vi "test Duplicate.vi"(8 "error in (no error)":errorcluster, 11 "TestCase In":refnum<class "Data Manipulation Tests.lvclass">) -> (0 "error out":errorcluster, 3 "TestCase Out":refnum<class "Data Manipulation Tests.lvclass">)   [LabVIEW 2017, in "Pointer Tests.lvlib" / "Data Manipulation Tests.lvclass"]
uses:
  Data Manipulation Tests.lvclass
  Source/Classes/Pointer/Pointer.lvclass/Pointer.ctl
  Source/Classes/Pointer/Public/New/New (4B).vi
  Source/Classes/Pointer/Public/Write/Write (1D I32).vi
  Source/Classes/Pointer/Private/Allocate.vi
  Source/Classes/Pointer/Public/Write (No Check)/Write (No Check 1D I32).vi
  Source/Classes/Pointer/Protected/Parameter Checking/Check Null Pointer.vi
  Source/Classes/Pointer/Protected/Parameter Checking/Check Subset (Power of 2).vi
  Source/Classes/Pointer/API/Accessors/Get Size.vi
  Source/Classes/Pointer/API/Copy All Pointer Data.vi
  Source/Classes/Pointer/Public/New/New (1B).vi
  Source/Classes/Pointer/Protected/Errors.vi
  Source/Classes/Pointer/Protected/Error VIs/Size Mismatch.vi
  Source/Classes/Pointer/API/Read Pointer Data.vi
  Source/Classes/Pointer/Public/Read/Read (1D U8).vi
  Source/Classes/Pointer/Private/Deallocate.vi
  Source/Classes/Pointer/API/Accessors/Set Address.vi
  Source/Classes/Pointer/API/Accessors/Set Size.vi
  Source/Classes/Pointer/Private/Set Internal.vi
  Source/Classes/Pointer/API/Accessors/Get Address.vi
  Source/Classes/Pointer/Protected/Error VIs/Null Pointer.vi
  Source/Classes/Pointer/Protected/Error VIs/Out of Bounds.vi
  Source/Classes/Pointer/Private/Count to Size.vi
  Source/Classes/Pointer/API/Copy Pointer Data.vi
  Source/Classes/Pointer/Protected/Error Building/Create Error.vi
  Source/VIs/Write String into Source.vi
  Source/VIs/Write Number into Source.vi
  Source/VIs/VIs for Poly/Write U64 into Source.vi
  Source/Classes/Pointer/Public/Read (No Check)/Read (No Check 1D U8).vi
  Source/Classes/Pointer/Protected/Get Internal.vi
  Source/Classes/Pointer/Protected/Error VIs/Zone.vi
  Source/Classes/Pointer/Protected/Error Building/Write Pointer Size.vi
  Source/Classes/Pointer/Public/Copy (No Check).vi
  Source/Classes/Pointer/Protected/Parameter Checking/Check Subset.vi
  Source/Constants/Constants.vi
  Source/Constants/Library Name.vi
  Source/Classes/Pointer/Protected/Error Building/Get Error Info.vi
  Source/VIs/Create Error Cluster.vi
  Source/VIs/VIs for Poly/Create Error Cluster (256B).vi
  Source/VIs/Set Error Status.vi
  Source/VIs/Set Error Code.vi
  Source/VIs/Set Error Source.vi
  Source/Classes/Pointer/Pointer.lvclass
  <vilib>/addons/_JKI Toolkits/VI Tester/TestCase.llb/TestCase.lvclass
  C:/Program Files (x86)/National Instruments/LabVIEW 2017/vi.lib/addons/_JKI Toolkits/VI Tester/TestCase.llb/TestCase.lvclass
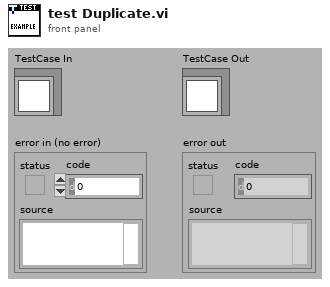
[diagram p1: front panel]
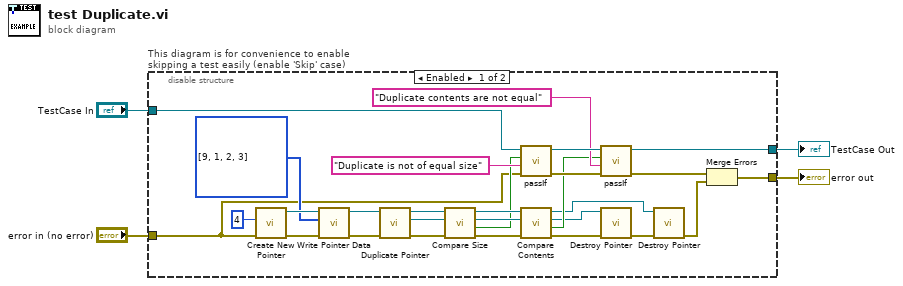
[diagram p0: block diagram]
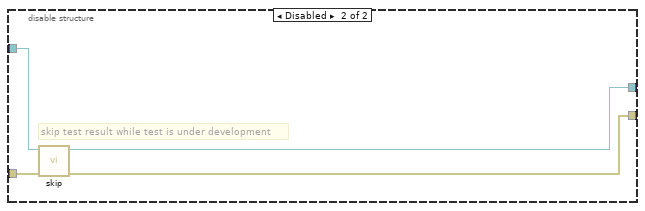
[diagram p2: hidden frame]
diagram:
  n1 = disable-structure "This diagram is for convenience to enable skipping a test easily (enable 'Skip' case)" shown="Enabled" {
    disable-tunnel: "TestCase In" -> [w30 w36]
    disable-tunnel: [w27 w34] -> w1
    disable-tunnel: [w11 w35] -> w3
    disable-tunnel: "error in (no error)" -> [w9 w33]
    frame Enabled {
      n2 = call-poly "Create New Pointer.vi"("error in (no error)"=w9, "count (1)"=u64 4) -> ("error out"=w15:errorcluster, "Pointer"=w32:refnum<class "Pointer.lvclass">)  [unwired: 8 in]
      n3 = call-poly "Write Pointer Data.vi"("error in (no error)"=w15, "buffer in"=i32[] [9, 1, 2, 3] ("count (1)"), "Pointer in"=w32) -> ("error out"=w14:errorcluster, "Pointer out"=w16:refnum<class "Pointer.lvclass">)  [unwired: 5 in, 2 out]
      n4 = call "Duplicate Pointer.vi"("error in (no error)"=w14, "Pointer in"=w16) -> ("error out"=w23:errorcluster, "new duplicate Pointer"=w20:refnum<class "Pointer.lvclass">, "Pointer out"=w24:refnum<class "Pointer.lvclass">)  [unwired: 7 in]
      n5 = call "Compare Size.vi"("error in (no error)"=w23, "Pointer b in"=w20, "Pointer a in"=w24) -> ("error out"=w21:errorcluster, "equal size?"=w18:bool, "Pointer b out"=w19:refnum<class "Pointer.lvclass">, "Pointer a out"=w22:refnum<class "Pointer.lvclass">)  [unwired: 5 in]
      n6 = call-dynamic "passIf.vi"("error in (no error)"=w9, "message (\"\")"="Duplicate is not of equal size" ("message (\"\")"), "pass"=w18, "TestCase in"=w30) -> ("error out"=w31:errorcluster, "TestCase out"=w28:refnum<class "Data Manipulation Tests.lvclass">)  [unwired: 6 in]
      n7 = call "Compare Contents.vi"("error in (no error)"=w21, "Pointer b in"=w19, "Pointer a in"=w22) -> ("error out"=w10:errorcluster, "equal contents?"=w17:bool, "Pointer b out"=w6:refnum<class "Pointer.lvclass">, "Pointer a out"=w5:refnum<class "Pointer.lvclass">)  [unwired: 5 in]
      n8 = call-dynamic "passIf.vi"("error in (no error)"=w31, "message (\"\")"="Duplicate contents are not equal" ("message (\"\")"), "pass"=w17, "TestCase in"=w28) -> ("error out"=w29:errorcluster, "TestCase out"=w27:refnum<class "Data Manipulation Tests.lvclass">)  [unwired: 6 in]
      n9 = call "Destroy Pointer.vi"("error in (no error)"=w10, "Pointer in"=w6) -> ("error out"=w8:errorcluster)  [unwired: 8 in, 1 out]
      n10 = call "Destroy Pointer.vi"("error in (no error)"=w8, "Pointer in"=w5) -> ("error out"=w7:errorcluster)  [unwired: 8 in, 1 out]
      n11 = Merge Errors(w29, w7) -> (w11:errorcluster)
    }
    frame Disabled {
      # "skip test result while test is under development"
      n12 = call <vilib>:"skip.vi"("error in (no error)"=w33, "TestCase in"=w36) -> ("error out"=w35:errorcluster, "TestCase out"=w34:refnum<class "Data Manipulation Tests.lvclass">)  [unwired: 8 in]
    }
  }
  "error out" <- w3
  "TestCase Out" <- w1
